vi "okCFrontPanel Read From Block Pipe Out.vi"(6 "Length":i32, 8 "Error In":errorcluster, 9 "Block Size":i32, 10 "Endpoint Addr":i32, 11 "okCFrontPanel Refnum":refnum<k24>) -> (0 "Error Out":errorcluster, 1 "BYTEARRAY":u8[](array[numeric]), 2 "ReadFromBlockPipeOut":i32, 3 "okCFrontPanel Refnum":refnum<k24>)   [LabVIEW 2019, in "okFrontPanelC#Wrapper.lvlib"]
uses:
  okFrontPanelC#Wrapper.lvlib
  C:/UCLA Thinkpad Google Drive/LabVIEW 2019 SP1/builds/SS2 Live Distribution/Opal Kelly/C# Wrapper/libFrontPanel-csharp.dll
  libFrontPanel-csharp.dll
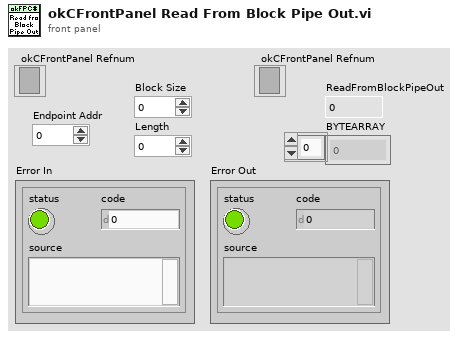
[diagram p1: front panel]
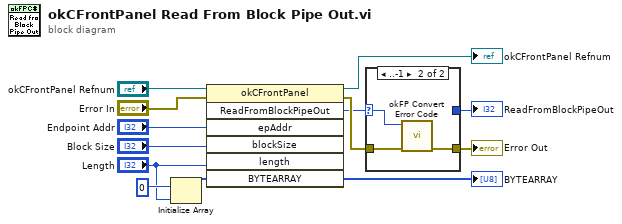
[diagram p0: block diagram]
diagram:
  n1 = Initialize Array(u8 0 ("BYTEARRAY"), "Length") -> (w6:u8[])
  n2 = invoke class="okCFrontPanel" method="ReadFromBlockPipeOut"(reference="okCFrontPanel Refnum", error in="Error In", "epAddr"="Endpoint Addr", "blockSize"="Block Size", "length"="Length", "BYTEARRAY"=w6) -> (reference out=→"okCFrontPanel Refnum":refnum<k24>, error out=w5:errorcluster, "ReadFromBlockPipeOut"=w3:i32, "BYTEARRAY"=→"BYTEARRAY":u8[])  [unwired: 1 in, 3 out]
  n3 = case shown="..-1" w3 {
    selector: w3 -> [w14 w16]
    tunnel: w5 -> [w15 w18]
    tunnel: [w15 w17] -> w4
    tunnel: [w14 _] -> w2
    frame 0, Default {
    }
    frame ..-1 {
      n4 = call "okFP Convert Error Code.vi"("error in (no error)"=w18, "okFP Error Code"=w16) -> ("error out"=w17:errorcluster)  [unwired: 9 in]
    }
  }
  "Error Out" <- w4
  "ReadFromBlockPipeOut" <- w2
